vi "Open Connection.vi"() -> ()   [LabVIEW 2017, in "LabSSH2.lvlib"]
uses:
  LabSSH2.lvlib
panel:
  in  "Address":string
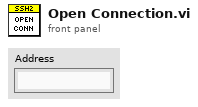
[diagram p1: front panel]
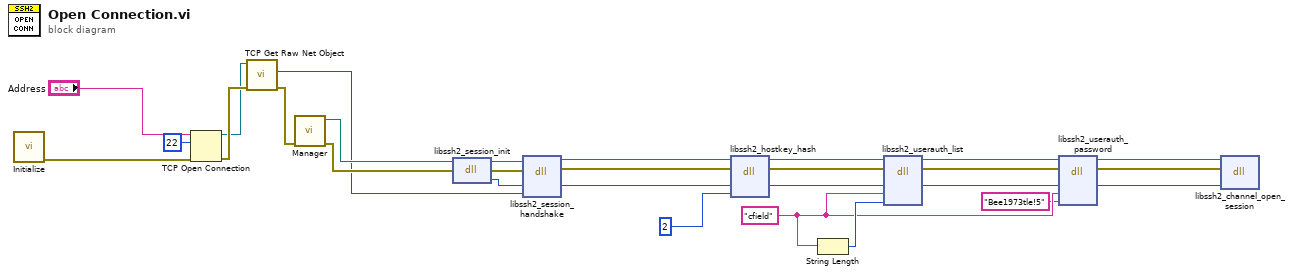
[diagram p0: block diagram]
diagram:
  w5 = "cfield" ("username")
  n1 = call "Initialize.vi"() -> ("Error Out"=w28:errorcluster)  [unwired: 11 in]
  n2 = TCP Open Connection(address="Address", remote port or service name=u16 22, error in (no error)=w28) -> (connection ID=w18:refnum<k5>, error out=w20:errorcluster)  [unwired: 2 in]
  n3 = call <vilib>:"TCP Get Raw Net Object.vi"("error in (no error)"=w20, "connection ID"=w18) -> ("error out"=w19:errorcluster, "raw net object"=w17:u64)  [unwired: 7 in, 1 out]
  n4 = call "Manager.vi"("Error In"=w19) -> ("Error Out"=w25:errorcluster, "Shared Library Out"=w24:path)  [unwired: 9 in]
  n5 = dll-call lib="D:/Users/cfield/Code/Field R&D Services/SSH/LabSSH2/LabVIEW/trunk/src/LabSSH2/Private/libssh2.*" fn="libssh2_session_init"(path in=w24, error in=w25) -> (path out=w23:path, error out=w22:errorcluster, "SESSION"=w21:i64)  [unwired: 1 in]
  n6 = dll-call lib="D:/Users/cfield/Code/Field R&D Services/SSH/LabSSH2/LabVIEW/trunk/src/LabSSH2/Private/libssh2.*" fn="libssh2_session_handshake"(path in=w23, error in=w22, "session"=w21, "socket"=w17) -> (path out=w15:path, error out=w16:errorcluster, "session"=w14:i64)  [unwired: 3 in]
  n7 = dll-call lib="D:/Users/cfield/Code/Field R&D Services/SSH/LabSSH2/LabVIEW/trunk/src/LabSSH2/Private/libssh2.*" fn="libssh2_hostkey_hash"(path in=w15, error in=w16, "session"=w14, "hash_type"=2) -> (path out=w11:path, error out=w12:errorcluster, "session"=w10:i64)  [unwired: 3 in]
  n8 = String Length(string=w5) -> (length=w9:i32)
  n9 = dll-call lib="D:/Users/cfield/Code/Field R&D Services/SSH/LabSSH2/LabVIEW/trunk/src/LabSSH2/Private/libssh2.*" fn="libssh2_userauth_list"(path in=w11, error in=w12, "session"=w10, "username"=w5, "username_len"=w9) -> (path out=w8:path, error out=w7:errorcluster, "session"=w6:i64)  [unwired: 4 in]
  n10 = dll-call lib="D:/Users/cfield/Code/Field R&D Services/SSH/LabSSH2/LabVIEW/trunk/src/LabSSH2/Private/libssh2.*" fn="libssh2_userauth_password"(path in=w8, error in=w7, "session"=w6, "username"=w5, "password"="Bee1973tle!5") -> (path out=w2:path, error out=w3:errorcluster, "session"=w1:i64)  [unwired: 4 in]
  n11 = dll-call lib="D:/Users/cfield/Code/Field R&D Services/SSH/LabSSH2/LabVIEW/trunk/src/LabSSH2/Private/libssh2.*" fn="libssh2_channel_open_session"(path in=w2, error in=w3, "session"=w1) -> ()  [unwired: 3 in, 2 out]
